vi "ELVIS III v1.0 Build MUX Configuration DI Block.vi"(11 "DI (N Samples) Channel List":T4) -> (0 "Configuration Bitmask Array":bool[][](array[boolean]), 1 "Configration Bitcode Array":bool[][](array[boolean]), 2 "DIO Mode Bitask":bool[][](array[boolean]), 3 "Channel Reservation List":T1)   [LabVIEW 2021]
uses:
  <vilib>/myRIO/Common/Instrument Driver Framework/myRIO v1.0/DI Block/typedefs/DI Block Channels List.ctl
  <vilib>/myRIO/Common/Instrument Driver Framework/myRIO v1.0/DI Block/typedefs/DI Block Channels Enum.ctl
  <vilib>/myRIO/Common/Instrument Driver Framework/ELVIS III v1.0/Resource Manager/typedefs/ELVIS III v1.0 Channel Reservation List.ctl
  <vilib>/myRIO/Common/Instrument Driver Framework/ELVIS III v1.0/Resource Manager/typedefs/ELVIS III v1.0 Channel Reservation Info.ctl
  <vilib>/myRIO/Common/Instrument Driver Framework/ELVIS III v1.0/Resource Manager/typedefs/ELVIS III v1.0 Connector List.ctl
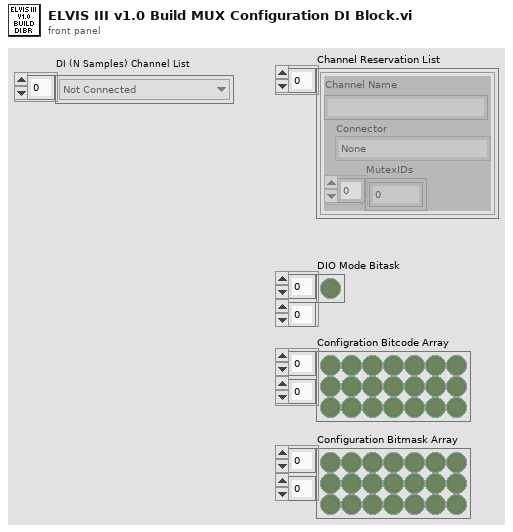
[diagram p1: front panel]
types:
  T1 = typedef "ELVIS III v1.0 Channel Reservation List.ctl" = T2[]
  T2 = typedef "ELVIS III v1.0 Channel Reservation Info.ctl" = cluster{"Channel Name":string, "Connector":T3, "MutexIDs":u32[]}
  T3 = typedef "ELVIS III v1.0 Connector List.ctl" = enum32{"None", "ConnectorA", "ConnectorB"}
  T4 = typedef "DI Block Channels List.ctl" = T5[]
  T5 = typedef "DI Block Channels Enum.ctl" = enum16{"Not Connected", "A/DI0 (N Samples)", "A/DI1 (N Samples)", "A/DI2 (N Samples)", "A/DI3 (N Samples)", "A/DI4 (N Samples)", "A/DI5 (N Samples)", "A/DI6 (N Samples)", "A/DI7 (N Samples)", "A/DI8 (N Samples)", "A/DI9 (N Samples)", "A/DI10 (N Samples)", "A/DI11 (N Samples)", "A/DI12 (N Samples)", "A/DI13 (N Samples)", "A/DI14 (N Samples)", "A/DI15 (N Samples)", "A/DI16 (N Samples)", "A/DI17 (N Samples)", "A/DI18 (N Samples)", "A/DI19 (N Samples)", "B/DI0 (N Samples)", "B/DI1 (N Samples)", "B/DI2 (N Samples)", "B/DI3 (N Samples)", "B/DI4 (N Samples)", "B/DI5 (N Samples)", "B/DI6 (N Samples)", "B/DI7 (N Samples)", "B/DI8 (N Samples)", "B/DI9 (N Samples)", "B/DI10 (N Samples)", "B/DI11 (N Samples)", "B/DI12 (N Samples)", "B/DI13 (N Samples)", "B/DI14 (N Samples)", "B/DI15 (N Samples)", "B/DI16 (N Samples)", "B/DI17 (N Samples)", "B/DI18 (N Samples)", "B/DI19 (N Samples)"}
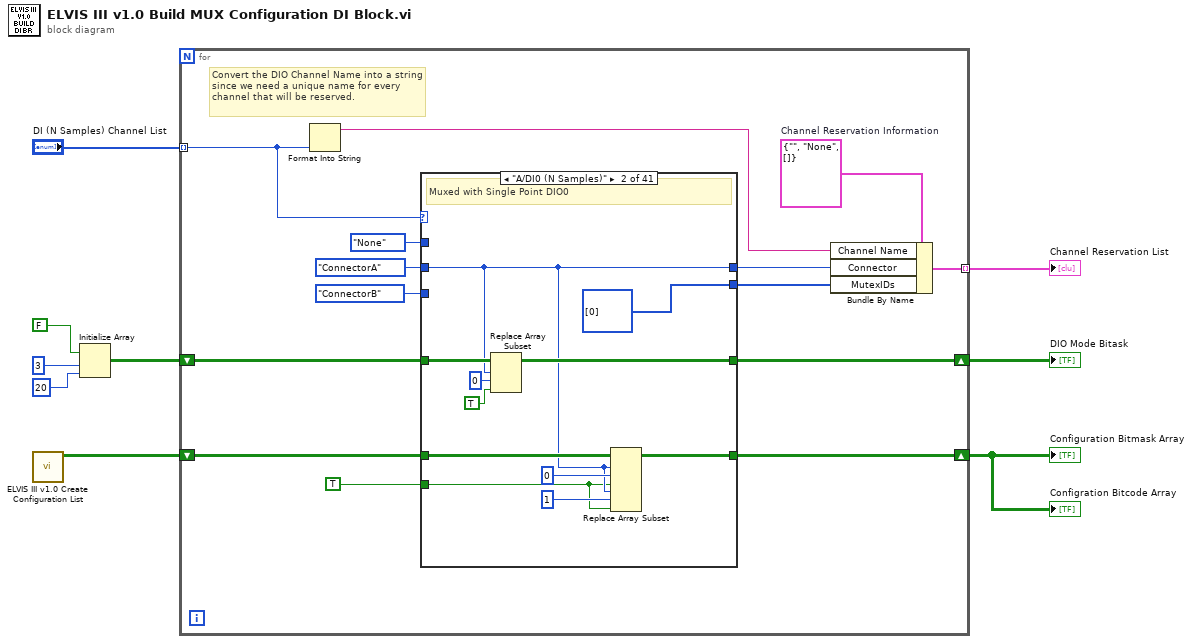
[diagram p0: block diagram]
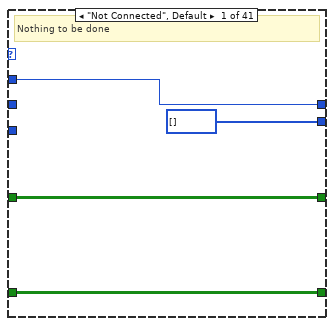
[diagram p2: hidden frame]
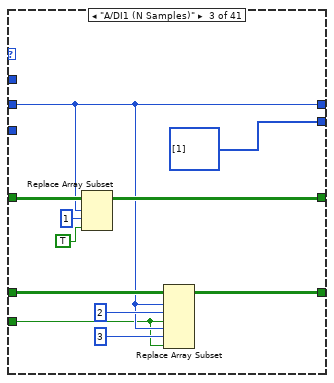
[diagram p3: hidden frame]
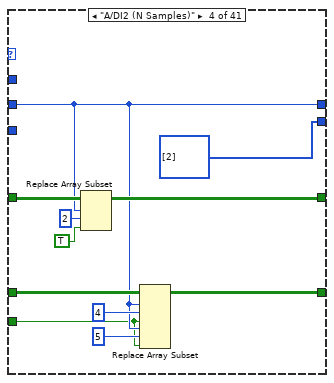
[diagram p4: hidden frame]
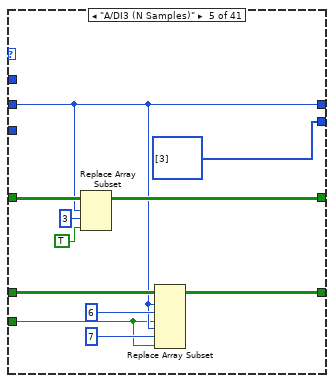
[diagram p5: hidden frame]
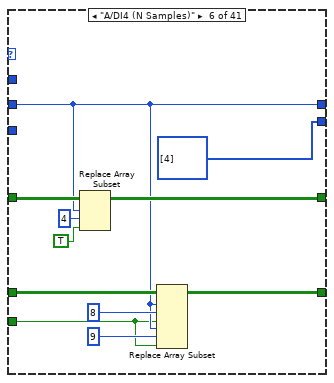
[diagram p6: hidden frame]
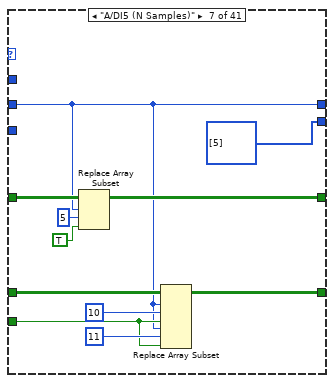
[diagram p7: hidden frame]
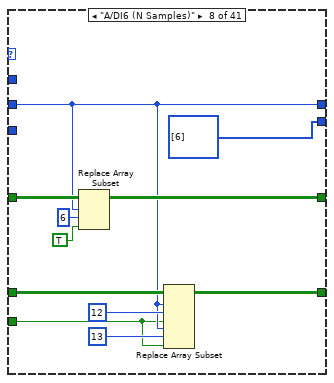
[diagram p8: hidden frame]
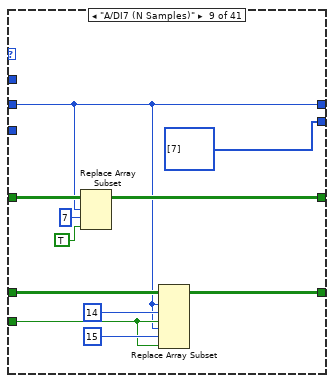
[diagram p9: hidden frame]
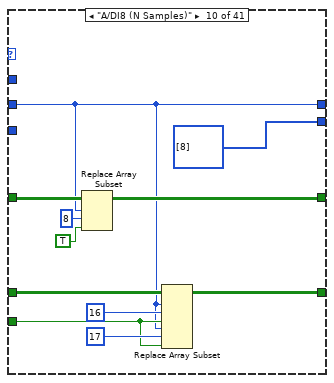
[diagram p10: hidden frame]
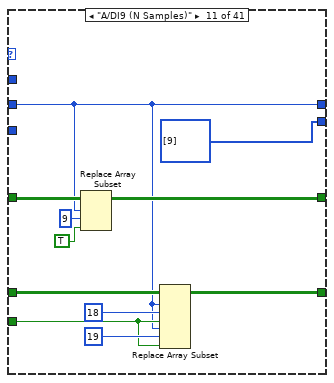
[diagram p11: hidden frame]
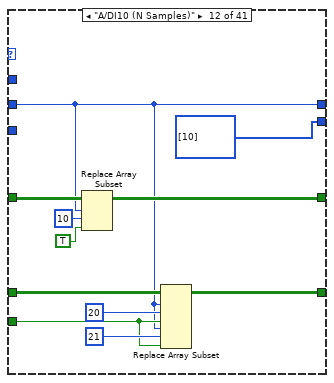
[diagram p12: hidden frame]
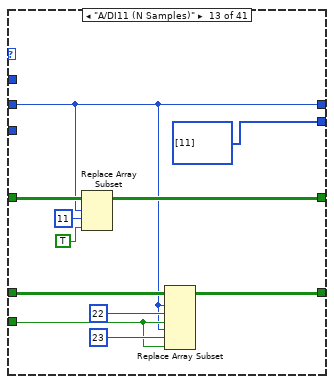
[diagram p13: hidden frame]
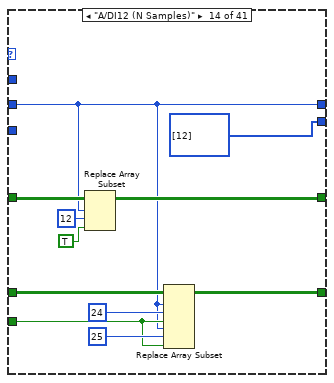
[diagram p14: hidden frame]
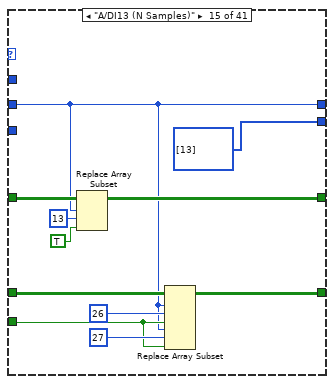
[diagram p15: hidden frame]
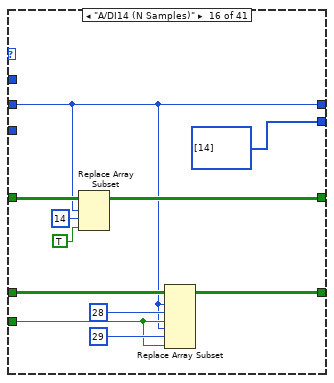
[diagram p16: hidden frame]
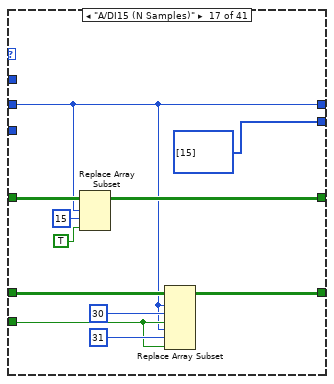
[diagram p17: hidden frame]
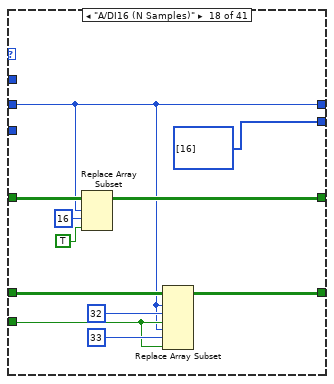
[diagram p18: hidden frame]
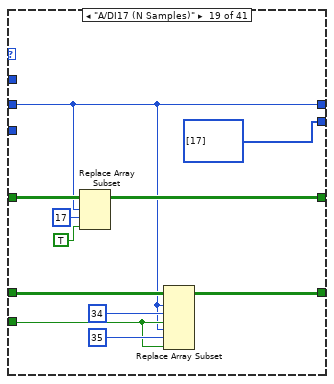
[diagram p19: hidden frame]
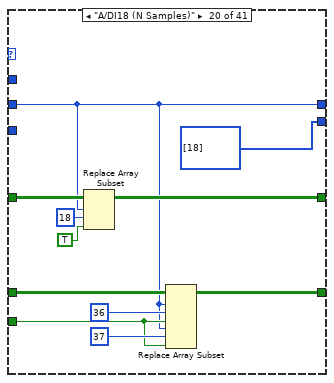
[diagram p20: hidden frame]
diagram:
  n1 = call <vilib>:"ELVIS III v1.0 Create Configuration List.vi"() -> ("Bitmask Array"=w2:bool[][])  [unwired: 11 in]
  n2 = Initialize Array(FALSE, 3 ("dimension size"), 20 ("dimension size")) -> (w4:bool[][])
  n3 = for {
    tunnel: "DI (N Samples) Channel List" -> [w17] mode=indexing
    tunnel: [w18] -> w8 mode=indexing
    shift-right: [w13] -> w3
    shift-left: w4 -> [w14]
    shift-right: [w10] -> w1
    shift-left: w2 -> [w12]
    w21 = T2 {"Channel Name"="", "Connector"=enum."None", "MutexIDs"=[]}  # Channel Reservation Information
    # "Convert the DIO Channel Name into a string since we need a unique name for every channel that will be reserved."
    n4 = Format Into String(w17) -> (resulting string=w16:string)  [unwired: 3 in, 1 out]
    n5 = case shown="\"A/DI0 (N Samples)\"" w17 {
      tunnel: ELVIS_III_v1.0_Connector_List."None" ("Connector List") -> [w27 _ _ _ _ _ _ _ _ _ _ _ _ _ _ _ _ _ _ _ _ _ _ _ _ _ _ _ _ _ _ _ _ _ _ _ _ _ _ _ _]
      tunnel: ELVIS_III_v1.0_Connector_List."ConnectorA" ("Connector List") -> [_ w30 w41 w52 w63 w74 w84 w96 w106 w117 w128 w139 w150 w161 w172 w183 w194 w205 w216 w227 w238 _ _ _ _ _ _ _ _ _ _ _ _ _ _ _ _ _ _ _ _]
      tunnel: [i32[] [] i32[] [0] i32[] [1] i32[] [2] i32[] [3] i32[] [4] i32[] [5] i32[] [6] i32[] [7] i32[] [8] i32[] [9] i32[] [10] i32[] [11] i32[] [12] i32[] [13] i32[] [14] i32[] [15] i32[] [16] i32[] [17] i32[] [18] i32[] [19] i32[] [0] i32[] [1] i32[] [2] i32[] [3] i32[] [4] i32[] [5] i32[] [6] i32[] [7] i32[] [8] i32[] [9] i32[] [10] i32[] [11] i32[] [12] i32[] [13] i32[] [14] i32[] [15] i32[] [16] i32[] [17] i32[] [18] i32[] [19]] -> w19
      tunnel: [w27 w30 w41 w52 w63 w74 w84 w96 w106 w117 w128 w139 w150 w161 w172 w183 w194 w205 w216 w227 w238 w249 w260 w271 w281 w293 w304 w315 w326 w337 w348 w359 w370 w381 w391 w403 w414 w425 w435 w447 w457] -> w20
      tunnel: ELVIS_III_v1.0_Connector_List."ConnectorB" ("Connector List") -> [_ _ _ _ _ _ _ _ _ _ _ _ _ _ _ _ _ _ _ _ _ w249 w260 w271 w281 w293 w304 w315 w326 w337 w348 w359 w370 w381 w391 w403 w414 w425 w435 w447 w457]
      tunnel: w14 -> [w25 w37 w46 w56 w68 w79 w90 w101 w111 w122 w133 w145 w155 w167 w177 w189 w200 w211 w222 w232 w244 w256 w265 w276 w287 w298 w310 w321 w332 w343 w354 w364 w376 w387 w397 w408 w420 w431 w441 w452 w463]
      tunnel: [w25 w36 w45 w57 w67 w78 w89 w100 w112 w123 w134 w144 w156 w166 w178 w188 w199 w210 w221 w233 w243 w254 w266 w277 w288 w299 w309 w320 w331 w342 w353 w365 w375 w386 w398 w409 w419 w430 w442 w453 w464] -> w13
      tunnel: w12 -> [w24 w31 w42 w53 w64 w75 w86 w97 w108 w119 w130 w141 w152 w163 w174 w185 w196 w207 w218 w229 w240 w251 w262 w273 w284 w295 w306 w317 w328 w339 w350 w361 w372 w383 w394 w405 w416 w427 w438 w449 w460]
      tunnel: TRUE ("new element/subarray") -> [_ w29 w40 w51 w62 w73 w85 w95 w107 w118 w129 w140 w151 w162 w173 w184 w195 w206 w217 w228 w239 w250 w261 w272 w283 w294 w305 w316 w327 w338 w349 w360 w371 w382 w393 w404 w415 w426 w437 w448 w459]
      tunnel: [w24 w28 w39 w50 w61 w72 w83 w94 w105 w116 w127 w138 w149 w160 w171 w182 w193 w204 w215 w226 w237 w248 w259 w270 w282 w292 w303 w314 w325 w336 w347 w358 w369 w380 w392 w402 w413 w424 w436 w446 w458] -> w10
      frame "Not Connected", Default {
        # "Nothing to be done"
      }
      frame "A/DI0 (N Samples)" {
        # "Muxed with Single Point DIO0"
        n6 = Replace Array Subset(array=w37, new element=TRUE ("new element/subarray"), index (row)=w30, index (col)=0 ("disabled index (col)")) -> (w36:bool[][])
        n7 = Replace Array Subset(array=w31, new element #1=w29, index (row) #1=w30, index (col) #1=0 ("disabled index (col)"), new element #2=w29, index (row) #2=w30, index (col) #2=1 ("disabled index (col)")) -> (w28:bool[][])
      }
      frame "A/DI1 (N Samples)" {
        n8 = Replace Array Subset(array=w46, new element=TRUE ("new element/subarray"), index (row)=w41, index (col)=1 ("disabled index (col)")) -> (w45:bool[][])
        n9 = Replace Array Subset(array=w42, new element #1=w40, index (row) #1=w41, index (col) #1=2 ("disabled index (col)"), new element #2=w40, index (row) #2=w41, index (col) #2=3 ("disabled index (col)")) -> (w39:bool[][])
      }
      frame "A/DI2 (N Samples)" {
        n10 = Replace Array Subset(array=w56, new element=TRUE ("new element/subarray"), index (row)=w52, index (col)=2 ("disabled index (col)")) -> (w57:bool[][])
        n11 = Replace Array Subset(array=w53, new element #1=w51, index (row) #1=w52, index (col) #1=4 ("disabled index (col)"), new element #2=w51, index (row) #2=w52, index (col) #2=5 ("disabled index (col)")) -> (w50:bool[][])
      }
      frame "A/DI3 (N Samples)" {
        n12 = Replace Array Subset(array=w68, new element=TRUE ("new element/subarray"), index (row)=w63, index (col)=3 ("disabled index (col)")) -> (w67:bool[][])
        n13 = Replace Array Subset(array=w64, new element #1=w62, index (row) #1=w63, index (col) #1=6 ("disabled index (col)"), new element #2=w62, index (row) #2=w63, index (col) #2=7 ("disabled index (col)")) -> (w61:bool[][])
      }
      frame "A/DI4 (N Samples)" {
        n14 = Replace Array Subset(array=w79, new element=TRUE ("new element/subarray"), index (row)=w74, index (col)=4 ("disabled index (col)")) -> (w78:bool[][])
        n15 = Replace Array Subset(array=w75, new element #1=w73, index (row) #1=w74, index (col) #1=8 ("disabled index (col)"), new element #2=w73, index (row) #2=w74, index (col) #2=9 ("disabled index (col)")) -> (w72:bool[][])
      }
      frame "A/DI5 (N Samples)" {
        n16 = Replace Array Subset(array=w90, new element=TRUE ("new element/subarray"), index (row)=w84, index (col)=5 ("disabled index (col)")) -> (w89:bool[][])
        n17 = Replace Array Subset(array=w86, new element #1=w85, index (row) #1=w84, index (col) #1=10 ("disabled index (col)"), new element #2=w85, index (row) #2=w84, index (col) #2=11 ("disabled index (col)")) -> (w83:bool[][])
      }
      frame "A/DI6 (N Samples)" {
        n18 = Replace Array Subset(array=w101, new element=TRUE ("new element/subarray"), index (row)=w96, index (col)=6 ("disabled index (col)")) -> (w100:bool[][])
        n19 = Replace Array Subset(array=w97, new element #1=w95, index (row) #1=w96, index (col) #1=12 ("disabled index (col)"), new element #2=w95, index (row) #2=w96, index (col) #2=13 ("disabled index (col)")) -> (w94:bool[][])
      }
      frame "A/DI7 (N Samples)" {
        n20 = Replace Array Subset(array=w111, new element=TRUE ("new element/subarray"), index (row)=w106, index (col)=7 ("disabled index (col)")) -> (w112:bool[][])
        n21 = Replace Array Subset(array=w108, new element #1=w107, index (row) #1=w106, index (col) #1=14 ("disabled index (col)"), new element #2=w107, index (row) #2=w106, index (col) #2=15 ("disabled index (col)")) -> (w105:bool[][])
      }
      frame "A/DI8 (N Samples)" {
        n22 = Replace Array Subset(array=w122, new element=TRUE ("new element/subarray"), index (row)=w117, index (col)=8 ("disabled index (col)")) -> (w123:bool[][])
        n23 = Replace Array Subset(array=w119, new element #1=w118, index (row) #1=w117, index (col) #1=16 ("disabled index (col)"), new element #2=w118, index (row) #2=w117, index (col) #2=17 ("disabled index (col)")) -> (w116:bool[][])
      }
      frame "A/DI9 (N Samples)" {
        n24 = Replace Array Subset(array=w133, new element=TRUE ("new element/subarray"), index (row)=w128, index (col)=9 ("disabled index (col)")) -> (w134:bool[][])
        n25 = Replace Array Subset(array=w130, new element #1=w129, index (row) #1=w128, index (col) #1=18 ("disabled index (col)"), new element #2=w129, index (row) #2=w128, index (col) #2=19 ("disabled index (col)")) -> (w127:bool[][])
      }
      frame "A/DI10 (N Samples)" {
        n26 = Replace Array Subset(array=w145, new element=TRUE ("new element/subarray"), index (row)=w139, index (col)=10 ("disabled index (col)")) -> (w144:bool[][])
        n27 = Replace Array Subset(array=w141, new element #1=w140, index (row) #1=w139, index (col) #1=20 ("disabled index (col)"), new element #2=w140, index (row) #2=w139, index (col) #2=21 ("disabled index (col)")) -> (w138:bool[][])
      }
      frame "A/DI11 (N Samples)" {
        n28 = Replace Array Subset(array=w155, new element=TRUE ("new element/subarray"), index (row)=w150, index (col)=11 ("disabled index (col)")) -> (w156:bool[][])
        n29 = Replace Array Subset(array=w152, new element #1=w151, index (row) #1=w150, index (col) #1=22 ("disabled index (col)"), new element #2=w151, index (row) #2=w150, index (col) #2=23 ("disabled index (col)")) -> (w149:bool[][])
      }
      frame "A/DI12 (N Samples)" {
        n30 = Replace Array Subset(array=w167, new element=TRUE ("new element/subarray"), index (row)=w161, index (col)=12 ("disabled index (col)")) -> (w166:bool[][])
        n31 = Replace Array Subset(array=w163, new element #1=w162, index (row) #1=w161, index (col) #1=24 ("disabled index (col)"), new element #2=w162, index (row) #2=w161, index (col) #2=25 ("disabled index (col)")) -> (w160:bool[][])
      }
      frame "A/DI13 (N Samples)" {
        n32 = Replace Array Subset(array=w177, new element=TRUE ("new element/subarray"), index (row)=w172, index (col)=13 ("disabled index (col)")) -> (w178:bool[][])
        n33 = Replace Array Subset(array=w174, new element #1=w173, index (row) #1=w172, index (col) #1=26 ("disabled index (col)"), new element #2=w173, index (row) #2=w172, index (col) #2=27 ("disabled index (col)")) -> (w171:bool[][])
      }
      frame "A/DI14 (N Samples)" {
        n34 = Replace Array Subset(array=w189, new element=TRUE ("new element/subarray"), index (row)=w183, index (col)=14 ("disabled index (col)")) -> (w188:bool[][])
        n35 = Replace Array Subset(array=w185, new element #1=w184, index (row) #1=w183, index (col) #1=28 ("disabled index (col)"), new element #2=w184, index (row) #2=w183, index (col) #2=29 ("disabled index (col)")) -> (w182:bool[][])
      }
      frame "A/DI15 (N Samples)" {
        n36 = Replace Array Subset(array=w200, new element=TRUE ("new element/subarray"), index (row)=w194, index (col)=15 ("disabled index (col)")) -> (w199:bool[][])
        n37 = Replace Array Subset(array=w196, new element #1=w195, index (row) #1=w194, index (col) #1=30 ("disabled index (col)"), new element #2=w195, index (row) #2=w194, index (col) #2=31 ("disabled index (col)")) -> (w193:bool[][])
      }
      frame "A/DI16 (N Samples)" {
        n38 = Replace Array Subset(array=w211, new element=TRUE ("new element/subarray"), index (row)=w205, index (col)=16 ("disabled index (col)")) -> (w210:bool[][])
        n39 = Replace Array Subset(array=w207, new element #1=w206, index (row) #1=w205, index (col) #1=32 ("disabled index (col)"), new element #2=w206, index (row) #2=w205, index (col) #2=33 ("disabled index (col)")) -> (w204:bool[][])
      }
      frame "A/DI17 (N Samples)" {
        n40 = Replace Array Subset(array=w222, new element=TRUE ("new element/subarray"), index (row)=w216, index (col)=17 ("disabled index (col)")) -> (w221:bool[][])
        n41 = Replace Array Subset(array=w218, new element #1=w217, index (row) #1=w216, index (col) #1=34 ("disabled index (col)"), new element #2=w217, index (row) #2=w216, index (col) #2=35 ("disabled index (col)")) -> (w215:bool[][])
      }
      frame "A/DI18 (N Samples)" {
        n42 = Replace Array Subset(array=w232, new element=TRUE ("new element/subarray"), index (row)=w227, index (col)=18 ("disabled index (col)")) -> (w233:bool[][])
        n43 = Replace Array Subset(array=w229, new element #1=w228, index (row) #1=w227, index (col) #1=36 ("disabled index (col)"), new element #2=w228, index (row) #2=w227, index (col) #2=37 ("disabled index (col)")) -> (w226:bool[][])
      }
      frame "A/DI19 (N Samples)" {
        n44 = Replace Array Subset(array=w244, new element=TRUE ("new element/subarray"), index (row)=w238, index (col)=19 ("disabled index (col)")) -> (w243:bool[][])
        n45 = Replace Array Subset(array=w240, new element #1=w239, index (row) #1=w238, index (col) #1=38 ("disabled index (col)"), new element #2=w239, index (row) #2=w238, index (col) #2=39 ("disabled index (col)")) -> (w237:bool[][])
      }
      frame "B/DI0 (N Samples)" {
        n46 = Replace Array Subset(array=w256, new element=TRUE ("new element/subarray"), index (row)=w249, index (col)=0 ("disabled index (col)")) -> (w254:bool[][])
        n47 = Replace Array Subset(array=w251, new element #1=w250, index (row) #1=w249, index (col) #1=0 ("disabled index (col)"), new element #2=w250, index (row) #2=w249, index (col) #2=1 ("disabled index (col)")) -> (w248:bool[][])
      }
      frame "B/DI1 (N Samples)" {
        n48 = Replace Array Subset(array=w265, new element=TRUE ("new element/subarray"), index (row)=w260, index (col)=1 ("disabled index (col)")) -> (w266:bool[][])
        n49 = Replace Array Subset(array=w262, new element #1=w261, index (row) #1=w260, index (col) #1=2 ("disabled index (col)"), new element #2=w261, index (row) #2=w260, index (col) #2=3 ("disabled index (col)")) -> (w259:bool[][])
      }
      frame "B/DI2 (N Samples)" {
        n50 = Replace Array Subset(array=w276, new element=TRUE ("new element/subarray"), index (row)=w271, index (col)=2 ("disabled index (col)")) -> (w277:bool[][])
        n51 = Replace Array Subset(array=w273, new element #1=w272, index (row) #1=w271, index (col) #1=4 ("disabled index (col)"), new element #2=w272, index (row) #2=w271, index (col) #2=5 ("disabled index (col)")) -> (w270:bool[][])
      }
      frame "B/DI3 (N Samples)" {
        n52 = Replace Array Subset(array=w287, new element=TRUE ("new element/subarray"), index (row)=w281, index (col)=3 ("disabled index (col)")) -> (w288:bool[][])
        n53 = Replace Array Subset(array=w284, new element #1=w283, index (row) #1=w281, index (col) #1=6 ("disabled index (col)"), new element #2=w283, index (row) #2=w281, index (col) #2=7 ("disabled index (col)")) -> (w282:bool[][])
      }
      frame "B/DI4 (N Samples)" {
        n54 = Replace Array Subset(array=w298, new element=TRUE ("new element/subarray"), index (row)=w293, index (col)=4 ("disabled index (col)")) -> (w299:bool[][])
        n55 = Replace Array Subset(array=w295, new element #1=w294, index (row) #1=w293, index (col) #1=8 ("disabled index (col)"), new element #2=w294, index (row) #2=w293, index (col) #2=9 ("disabled index (col)")) -> (w292:bool[][])
      }
      frame "B/DI5 (N Samples)" {
        n56 = Replace Array Subset(array=w310, new element=TRUE ("new element/subarray"), index (row)=w304, index (col)=5 ("disabled index (col)")) -> (w309:bool[][])
        n57 = Replace Array Subset(array=w306, new element #1=w305, index (row) #1=w304, index (col) #1=10 ("disabled index (col)"), new element #2=w305, index (row) #2=w304, index (col) #2=11 ("disabled index (col)")) -> (w303:bool[][])
      }
      frame "B/DI6 (N Samples)" {
        n58 = Replace Array Subset(array=w321, new element=TRUE ("new element/subarray"), index (row)=w315, index (col)=6 ("disabled index (col)")) -> (w320:bool[][])
        n59 = Replace Array Subset(array=w317, new element #1=w316, index (row) #1=w315, index (col) #1=12 ("disabled index (col)"), new element #2=w316, index (row) #2=w315, index (col) #2=13 ("disabled index (col)")) -> (w314:bool[][])
      }
      frame "B/DI7 (N Samples)" {
        n60 = Replace Array Subset(array=w332, new element=TRUE ("new element/subarray"), index (row)=w326, index (col)=7 ("disabled index (col)")) -> (w331:bool[][])
        n61 = Replace Array Subset(array=w328, new element #1=w327, index (row) #1=w326, index (col) #1=14 ("disabled index (col)"), new element #2=w327, index (row) #2=w326, index (col) #2=15 ("disabled index (col)")) -> (w325:bool[][])
      }
      frame "B/DI8 (N Samples)" {
        n62 = Replace Array Subset(array=w343, new element=TRUE ("new element/subarray"), index (row)=w337, index (col)=8 ("disabled index (col)")) -> (w342:bool[][])
        n63 = Replace Array Subset(array=w339, new element #1=w338, index (row) #1=w337, index (col) #1=16 ("disabled index (col)"), new element #2=w338, index (row) #2=w337, index (col) #2=17 ("disabled index (col)")) -> (w336:bool[][])
      }
      frame "B/DI9 (N Samples)" {
        n64 = Replace Array Subset(array=w354, new element=TRUE ("new element/subarray"), index (row)=w348, index (col)=9 ("disabled index (col)")) -> (w353:bool[][])
        n65 = Replace Array Subset(array=w350, new element #1=w349, index (row) #1=w348, index (col) #1=18 ("disabled index (col)"), new element #2=w349, index (row) #2=w348, index (col) #2=19 ("disabled index (col)")) -> (w347:bool[][])
      }
      frame "B/DI10 (N Samples)" {
        n66 = Replace Array Subset(array=w364, new element=TRUE ("new element/subarray"), index (row)=w359, index (col)=10 ("disabled index (col)")) -> (w365:bool[][])
        n67 = Replace Array Subset(array=w361, new element #1=w360, index (row) #1=w359, index (col) #1=20 ("disabled index (col)"), new element #2=w360, index (row) #2=w359, index (col) #2=21 ("disabled index (col)")) -> (w358:bool[][])
      }
      frame "B/DI11 (N Samples)" {
        n68 = Replace Array Subset(array=w376, new element=TRUE ("new element/subarray"), index (row)=w370, index (col)=11 ("disabled index (col)")) -> (w375:bool[][])
        n69 = Replace Array Subset(array=w372, new element #1=w371, index (row) #1=w370, index (col) #1=22 ("disabled index (col)"), new element #2=w371, index (row) #2=w370, index (col) #2=23 ("disabled index (col)")) -> (w369:bool[][])
      }
      frame "B/DI12 (N Samples)" {
        n70 = Replace Array Subset(array=w387, new element=TRUE ("new element/subarray"), index (row)=w381, index (col)=12 ("disabled index (col)")) -> (w386:bool[][])
        n71 = Replace Array Subset(array=w383, new element #1=w382, index (row) #1=w381, index (col) #1=24 ("disabled index (col)"), new element #2=w382, index (row) #2=w381, index (col) #2=25 ("disabled index (col)")) -> (w380:bool[][])
      }
      frame "B/DI13 (N Samples)" {
        n72 = Replace Array Subset(array=w397, new element=TRUE ("new element/subarray"), index (row)=w391, index (col)=13 ("disabled index (col)")) -> (w398:bool[][])
        n73 = Replace Array Subset(array=w394, new element #1=w393, index (row) #1=w391, index (col) #1=26 ("disabled index (col)"), new element #2=w393, index (row) #2=w391, index (col) #2=27 ("disabled index (col)")) -> (w392:bool[][])
      }
      frame "B/DI14 (N Samples)" {
        n74 = Replace Array Subset(array=w408, new element=TRUE ("new element/subarray"), index (row)=w403, index (col)=14 ("disabled index (col)")) -> (w409:bool[][])
        n75 = Replace Array Subset(array=w405, new element #1=w404, index (row) #1=w403, index (col) #1=28 ("disabled index (col)"), new element #2=w404, index (row) #2=w403, index (col) #2=29 ("disabled index (col)")) -> (w402:bool[][])
      }
      frame "B/DI15 (N Samples)" {
        n76 = Replace Array Subset(array=w420, new element=TRUE ("new element/subarray"), index (row)=w414, index (col)=15 ("disabled index (col)")) -> (w419:bool[][])
        n77 = Replace Array Subset(array=w416, new element #1=w415, index (row) #1=w414, index (col) #1=30 ("disabled index (col)"), new element #2=w415, index (row) #2=w414, index (col) #2=31 ("disabled index (col)")) -> (w413:bool[][])
      }
      frame "B/DI16 (N Samples)" {
        n78 = Replace Array Subset(array=w431, new element=TRUE ("new element/subarray"), index (row)=w425, index (col)=16 ("disabled index (col)")) -> (w430:bool[][])
        n79 = Replace Array Subset(array=w427, new element #1=w426, index (row) #1=w425, index (col) #1=32 ("disabled index (col)"), new element #2=w426, index (row) #2=w425, index (col) #2=33 ("disabled index (col)")) -> (w424:bool[][])
      }
      frame "B/DI17 (N Samples)" {
        n80 = Replace Array Subset(array=w441, new element=TRUE ("new element/subarray"), index (row)=w435, index (col)=17 ("disabled index (col)")) -> (w442:bool[][])
        n81 = Replace Array Subset(array=w438, new element #1=w437, index (row) #1=w435, index (col) #1=34 ("disabled index (col)"), new element #2=w437, index (row) #2=w435, index (col) #2=35 ("disabled index (col)")) -> (w436:bool[][])
      }
      frame "B/DI18 (N Samples)" {
        n82 = Replace Array Subset(array=w452, new element=TRUE ("new element/subarray"), index (row)=w447, index (col)=18 ("disabled index (col)")) -> (w453:bool[][])
        n83 = Replace Array Subset(array=w449, new element #1=w448, index (row) #1=w447, index (col) #1=36 ("disabled index (col)"), new element #2=w448, index (row) #2=w447, index (col) #2=37 ("disabled index (col)")) -> (w446:bool[][])
      }
      frame "B/DI19 (N Samples)" {
        n84 = Replace Array Subset(array=w463, new element=TRUE ("new element/subarray"), index (row)=w457, index (col)=19 ("disabled index (col)")) -> (w464:bool[][])
        n85 = Replace Array Subset(array=w460, new element #1=w459, index (row) #1=w457, index (col) #1=38 ("disabled index (col)"), new element #2=w459, index (row) #2=w457, index (col) #2=39 ("disabled index (col)")) -> (w458:bool[][])
      }
    }
    n86 = Bundle By Name(cluster=w21, "Channel Name"=w16, "Connector"=w20, "MutexIDs"=w19) -> (w18:T2)
  }
  "Channel Reservation List" <- w8
  "DIO Mode Bitask" <- w3
  "Configuration Bitmask Array" <- w1
  "Configration Bitcode Array" <- w1
